vi "testEventsSimple.vi"() -> ()   [LabVIEW 2017]
panel:
  out "number of events discarded":u32
  in  "ID":string="theid"
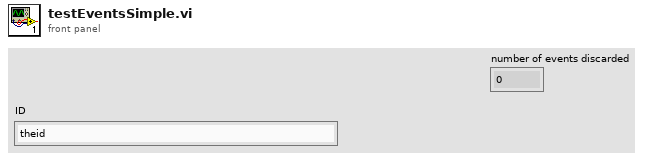
[diagram p1: front panel]
types:
  T1 = typedef "LVPortEventRegistrationDataType.ctl" = refnum<event-registration>
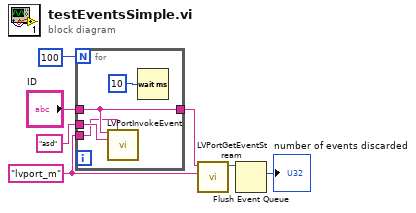
[diagram p0: block diagram]
diagram:
  w1 = "lvport_m" ("Category")
  n1 = for {
    N: 100 -> [_]
    tunnel: "asd" ("name") -> [w11]
    tunnel: "ID" -> [w10]
    tunnel: [w10] -> w2
    tunnel: w1 -> [w8]
    n2 = call "LVPortInvokeEvent.vi"("ID"=w10, "Category"=w8, "name"=w11) -> ()  [unwired: 12 in, 1 out]
    n3 = Wait (ms)(milliseconds to wait=u32 10) -> ()  [unwired: 1 out]
  }
  n4 = call "LVPortGetEventStream.vi"("Category"=w1, "ID"=w2) -> ("Event Registration Refnum out"=w4:T1)  [unwired: 6 in, 3 out]
  n5 = Flush Event Queue(0:w4) -> (9:→"number of events discarded":u32)  [unwired: 5 in, 2 out]
